vi "Display Images_.vi"(0 "fpga interface in":refnum<k20>, 1 "'stop' notifier":refnum<notifier>, 3 "measure call context in":refnum<class "Measure Call Context.lvclass">, 11 "error in (no error)":errorcluster, 12 "References":T1) -> (4 "fpga interface out":refnum<k20>, 15 "error out":errorcluster)   [LabVIEW 2025, in "GettingStarted_Common_148X_Host.lvlib"]
uses:
  GettingStarted_Common_148X_Host.lvlib
  <vilib>/Plug-In SDKs/Measurements/Measure Call Context/Measure Call Context.lvclass
  Types/148x_Common_FPGA_Reference.ctl
  <instrlib>/FlexRIO/CSI-2/v2/Common/Types/LLP Data Type.ctl
  Measurement Results.ctl
  <vilib>/Utility/error.llb/Error Cluster From Error Code.vi
  <vilib>/rvi/errors/niLvFpgaAdjustHostInterfaceError.vi
  <vilib>/rvi/interface/nirviReadWriteControl/nirviReadWriteControl.xnode
  NiFpgaLv.dll
  <vilib>/rvi/interface/Simulation/niFpgaSimulationCallBeginRW.vi
  Automotive Vision.lvclass
  <instrlib>/FlexRIO/CSI-2/v2/Common/NI CSI-2 API Common v2.lvlib
panel:
  in  "Image decimation":u32=5
  in  "Decimate image":bool
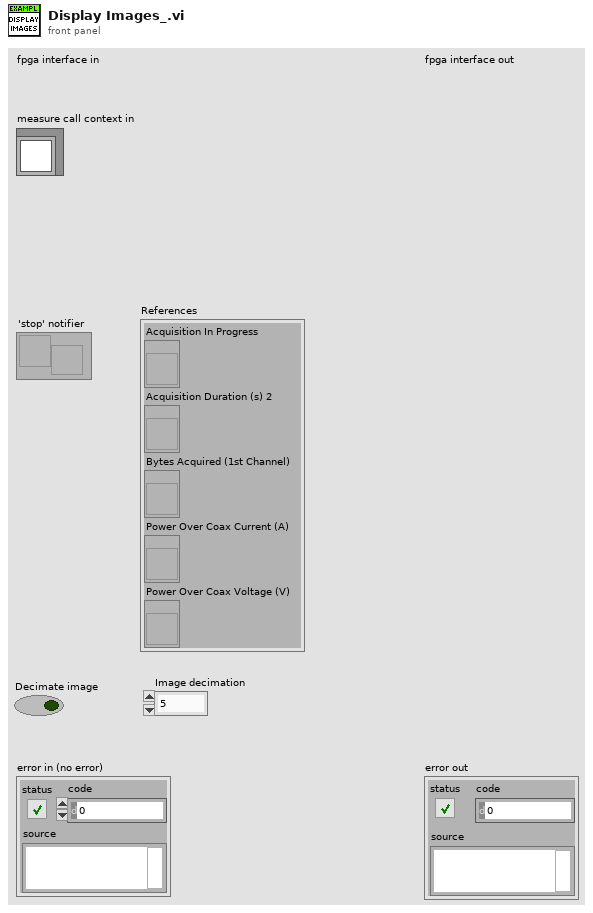
[diagram p1: front panel]
types:
  T1 = cluster{"Acquisition In Progress":refnum<vi>, "Acquisition Duration (s) 2":refnum<vi>, "Bytes Acquired (1st Channel)":refnum<vi>, "Power Over Coax Current (A)":refnum<vi>, "Power Over Coax Voltage (V)":refnum<vi>}
  T2 = typedef "NI CSI-2 API Common v2.lvlib/LLP Data Type.ctl" = enum8{"Frame Start", "Frame End", "Line Start", "Line End", "End of Transmission", "Reserved 0", "Reserved 1", "Reserved 2", "Generic Short Packet 1", "Generic Short Packet 2", "Generic Short Packet 3", "Generic Short Packet 4", "Generic Short Packet 5", "Generic Short Packet 6", "Generic Short Packet 7", "Generic Short Packet 8", "Null", "Blanking Data", "Embedded 8-bit non Image Data", "Generic Long Packet 1", "Generic Long Packet 2", "Generic Long Packet 3", "Generic Long Packet 4", "Reserved 3", "YUV420 8-bit", "YUV420 10-bit", "Legacy YUV420 8-bit", "Reserved 4", "YUV420 8-bit Chroma Shifted", "YUV420 10-bit Chroma Shifted", "YUV422 8-bit", "YUV422 10-bit", "RGB444", "RGB555", "RGB565", "RGB666", "RGB888", "Reserved 5", "Reserved 6", "RAW 24", "RAW 6", "RAW 7", "RAW 8", "RAW 10", "RAW 12", "RAW 14", "RAW 16", "RAW 20", "User Defined 8-bit Data 1", "User Defined 8-bit Data 2", "User Defined 8-bit Data 3", "User Defined 8-bit Data 4", "User Defined 8-bit Data 5", "User Defined 8-bit Data 6", "User Defined 8-bit Data 7", "User Defined 8-bit Data 8", "USL Command", "Reserved 7", "Reserved 8", "Reserved 9", "Reserved 10", "Reserved 11", "Reserved 12", "LRTE EPD Spacer"}
  T3 = cluster{"serial channel":fxp<+,3,3>, "frame number":u16, "data type":T2, "width":u16, "height":u16, "image bytes":u32, "total bytes":u32, "little endian":bool, "Status":string}
  T4 = typedef "GettingStarted_Common_148X_Host.lvlib/148x_Common_FPGA_Reference.ctl" = refnum<k20>
  T5 = typedef "Automotive Vision.lvclass/Measurement Results.ctl" = cluster{"ACQ. IN PROGRESS":bool, "Array":u32[], "ACQ. DURATION (s)":dbl, "SOURCE RATE (fps)":dbl, "BYTES ACQUIRED":u64, "FRAME COUNT":u64, "POC VOLTAGE (V)":dbl, "POC CURRENT (A)":dbl, "ERROR":bool, "STATE MESSAGE":string, "IMAGE DATA":string, "OOB gRPC Port":i32}
  T6 = typedef "GettingStarted_Common_148X_FPGA.lvlib/Image Metadata.ctl" = cluster{"serial channel":fxp<+,3,3>, "frame number":u16, "data type":T2, "width":u16, "height":u16, "image bytes":u32, "total bytes":u32, "little endian":bool}
  T7 = typedef "Automotive-Vision OOB Data Transfer.lvlib/OOB to Logic Data.ctl" = cluster{"PauseResume":bool, "ExportPath":string, "ExportType":u16, "Export":bool}
  T8 = cluster{"image pixel data fifo overflow":bool, "image metadata fifo overflow":bool}[]
  T9 = cluster{"image pixel data fifo overflow":bool, "image metadata fifo overflow":bool}
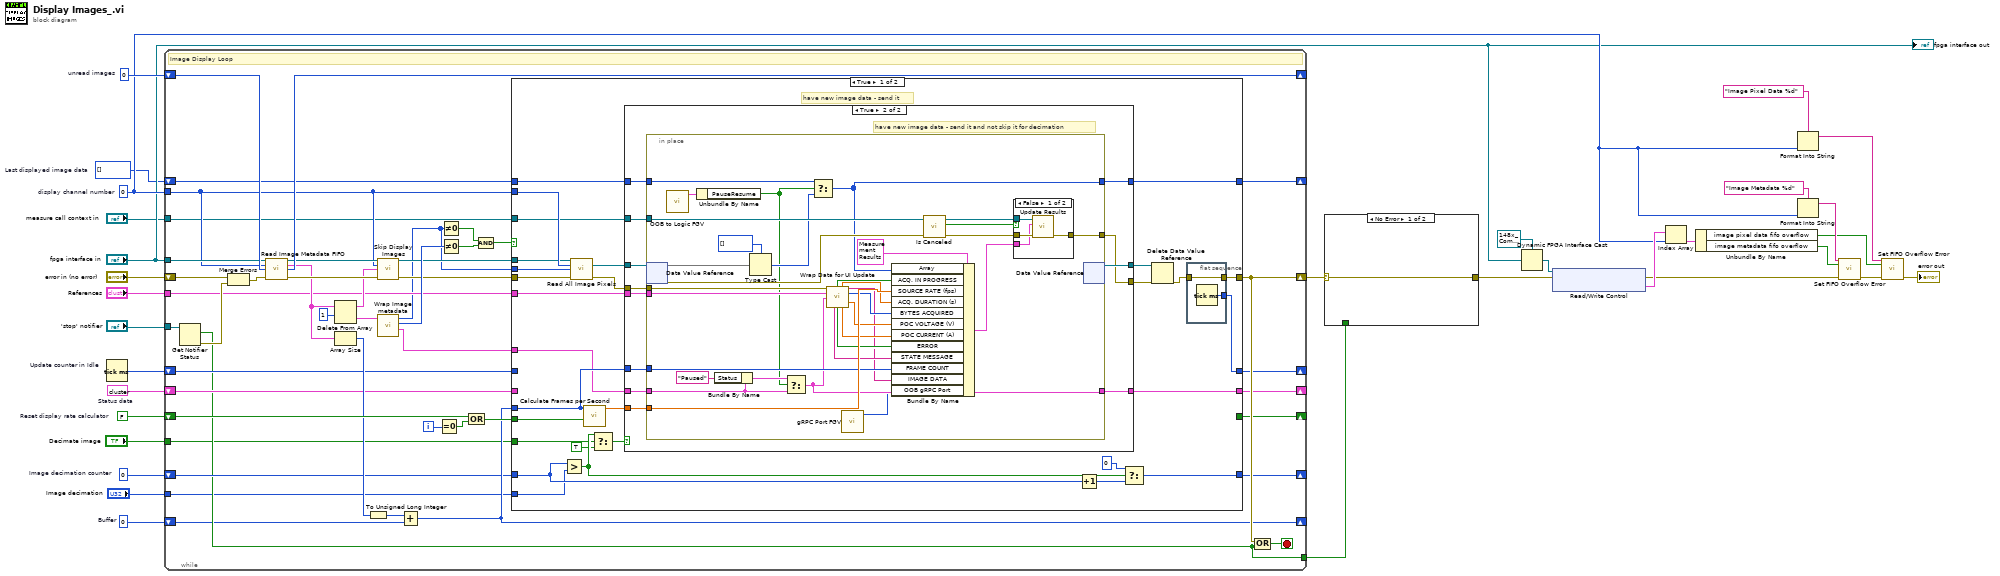
[diagram p0: block diagram]
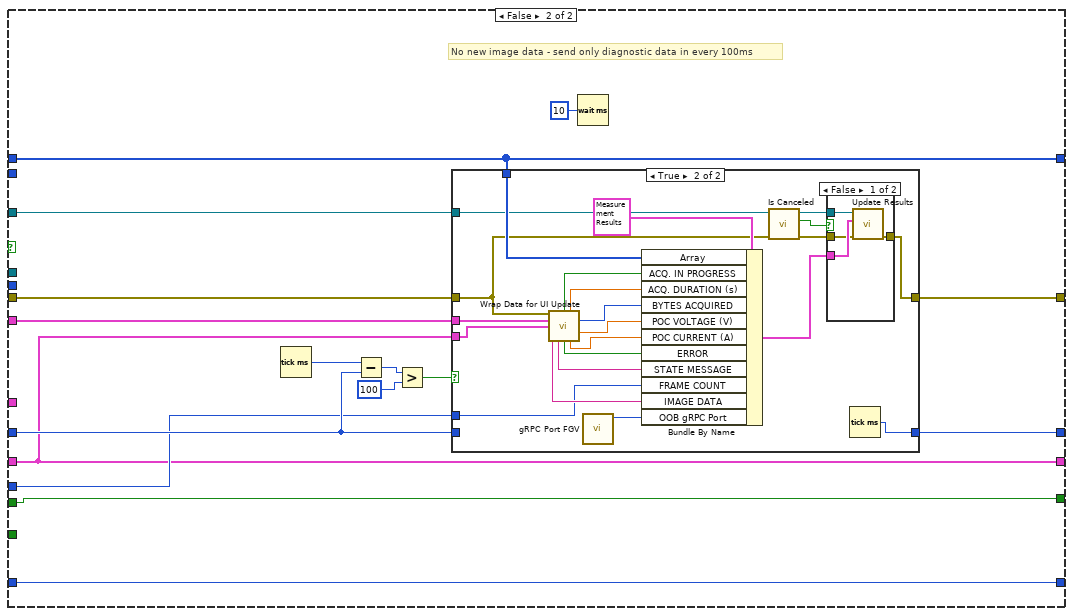
[diagram p4: hidden frame]
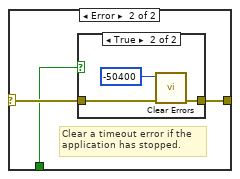
[diagram p7: hidden frame]
diagram:
  w3 = T3 {"serial channel"=0.0, "frame number"=0, "data type"=enum."Frame Start", "width"=0, "height"=0, "image bytes"=0, "total bytes"=0, "little endian"=FALSE, "Status"="Ready for Acquisition"}  # Status data
  w22 = 0  # display channel number
  w7 = u32 0  # Image decimation counter
  w8 = u32[] []  # Last displayed image data
  w14 = u32 0  # Buffer
  w15 = FALSE  # Reset display rate calculator
  w31 = u32 0  # unread images
  n1 = Tick Count (ms) "Update counter in Idle"() -> (millisecond timer value=w9:u32)
  n2 = while {
    shift-right: [w74] -> w13
    shift-left: "error in (no error)" -> [w50]
    tunnel: "fpga interface in" -> [w53]
    shift-right: [w75] -> _
    shift-left: w31 -> [w65]
    tunnel: w22 -> [w49]
    shift-right: [w69] -> _
    shift-left: w15 -> [w66]
    shift-right: [w55] -> _
    shift-left: w14 -> [w32]
    tunnel: [w36] -> w11
    tunnel: "'stop' notifier" -> [w52]
    shift-right: [w47] -> _
    shift-left: w9 -> [w48]
    shift-right: [w45] -> _
    shift-left: w8 -> [w46]
    shift-right: [w43] -> _
    shift-left: w7 -> [w44]
    tunnel: "References" -> [w42]
    tunnel: "measure call context in" -> [w41]
    shift-right: [w39] -> _
    shift-left: w3 -> [w40]
    tunnel: "Image decimation" -> [w35]
    tunnel: "Decimate image" -> [w34]
    i -> [w73]
    stop <- w76 stop-if-true
    # "Image Display Loop"
    n3 = Get Notifier Status(notifier=w52) -> (current notification=w36:bool, error out=w77:errorcluster)  [unwired: 1 in, 3 out]
    n4 = Merge Errors(w50, w77) -> (w51:errorcluster)
    n5 = call "Read Image Metadata FIFO.vi"("fpga inteface in"=w53, "display channel number"=w49, "number of images"=w65, "error in (no error)"=w51) -> ("fpga interface out"=w61:refnum<k20>, "image metadata"=w54:T6[], "images remaining"=w75:u32, "error out"=w58:errorcluster)  [unwired: 8 in]
    n6 = Delete From Array(array=w54, length=1) -> (deleted portion=w62:T6[], array with subset deleted=w57:T6[])  [unwired: 1 in]
    n7 = Array Size(array=w54) -> (size(s)=w56:i32)
    n8 = To Unsigned Long Integer(number=w56) -> (unsigned 32bit integer=w33:u32)
    n9 = call "Skip Display Images.vi"("fpga interface in"=w61, "display channel number"=w49, "image metadata"=w57, "error in (no error)"=w58) -> ("fpga interface out"=w60:refnum<k20>, "error out"=w59:errorcluster)  [unwired: 10 in]
    n10 = call "Wrap Image metadata.vi"("image metadata"=w62) -> ("element"=w38:T3, "Numeric"=w64:i32, "total bytes"=w37:u32)  [unwired: 8 in]
    n11 = Add(x=w33, y=w32) -> (x+y=w55:u32)
    n12 = Equal To 0?(x=w73) -> (x = 0?=w67:bool)
    n13 = Not Equal To 0?(x=w37) -> (x != 0?=w71:bool)
    n14 = Not Equal To 0?(x=w64) -> (x != 0?=w72:bool)
    n15 = Compound Arithmetic op=OR(w66, w67) -> (w68:bool)
    n16 = Compound Arithmetic op=AND(w71, w72) -> (w70:bool)
    n17 = case shown="True" w70 {
      tunnel: w59 -> [w102 w162]
      tunnel: w60 -> [w105 _]
      tunnel: w49 -> [w106 _]
      tunnel: [w96 w169] -> w74
      tunnel: w68 -> [w81 w176]
      tunnel: [_ w176] -> w69
      tunnel: w55 -> [w93 w166]
      tunnel: w37 -> [w100 _]
      tunnel: w38 -> [w84 _]
      tunnel: w41 -> [w98 w163]
      tunnel: w42 -> [w97 w177]
      tunnel: w48 -> [_ w168]
      tunnel: [w95 w170] -> w47
      tunnel: w46 -> [w92 w167]
      tunnel: [w94 w167] -> w45
      tunnel: w44 -> [w90 w165]
      tunnel: [w88 w165] -> w43
      tunnel: w40 -> [_ w164]
      tunnel: [w83 w164] -> w39
      tunnel: w35 -> [w79 _]
      tunnel: w34 -> [w78 _]
      frame True {
        # "have new image data - send it"
        n18 = Greater?(x=w90, y=w79) -> (0:w87:bool)
        n19 = call "Read All Image Pixels.vi"("fpga inteface in"=w105, "display channel number"=w106, "image bytes"=w100, "error in (no error)"=w102) -> ("image pixel data region"=w104:refnum<data-value>, "error out"=w99:errorcluster)  [unwired: 8 in, 2 out]
        n20 = call <vilib>:"Calculate Frames per Second.vi"("Reset"=w81, "Buffer Number"=w93) -> ("Acquired Frames/s"=w80:dbl)  [unwired: 7 in, 2 out]
        n21 = Select(t=w87, s=w78, f=TRUE) -> (s? t:f=w86:bool)
        n22 = case shown="True" w86 {
          tunnel: w104 -> [w110 w122]
          tunnel: [w110 w121] -> w103
          tunnel: [w108 w120] -> w101
          tunnel: w80 -> [_ w119]
          tunnel: w99 -> [w108 w118]
          tunnel: w84 -> [w107 w117]
          tunnel: w98 -> [_ w116]
          tunnel: w97 -> [_ w115]
          tunnel: [w109 w114] -> w94
          tunnel: w93 -> [_ w113]
          tunnel: w92 -> [w109 w112]
          tunnel: [w107 w111] -> w83
          frame False {
            # "have new image data - but skip the sending to not overload UI with data transfer"
          }
          frame True {
            # "have new image data - send it and not skip it for decimation"
            n23 = in-place {
              in-place-border: [w150] -> w120
              in-place-border: w119 -> [w149]
              in-place-border: w118 -> [w148]
              in-place-border: w117 -> [w147]
              in-place-border: w116 -> [w146]
              in-place-border: w115 -> [w145]
              in-place-border: [w144] -> w114
              in-place-border: w113 -> [w143]
              in-place-border: w112 -> [w142]
              in-place-border: [w141] -> w111
              n24 = in-place-dvr #1(w122) -> (w151:u8[], w153:errorcluster)
              n25 = call "OOB to Logic FGV.vi"() -> ("OOB to Logic Data out"=w124:T7)  [unwired: 10 in, 1 out]
              n26 = Unbundle By Name(w124) -> ("PauseResume"=w123:bool)
              n27 = Bundle By Name(cluster=w147, "Status"="Paused") -> (w128:T3)
              n28 = Type Cast(type=u32[] [], x=w151) -> (*(type *) &x=w129:u32[])
              n29 = Select(t=w128, s=w123, f=w147) -> (s? t:f=w141:T3)
              n30 = Select(t=w142, s=w123, f=w129) -> (s? t:f=w144:u32[])
              n31 = call "Wrap Data for UI Update.vi"("error in (no error)"=w148, "References"=w145, "image metadata"=w141) -> ("Acqusition In Progress"=w137:bool, "Acquisition Duration"=w136:dbl, "Image Data"=w130:string, "Bytes Acquired"=w135:i64, "PowerOverCoaxCurrent"=w134:dbl, "State message"=w131:string, "status"=w132:bool, "PowerOverCoaxVoltage"=w133:dbl)  [unwired: 4 in, 1 out]
              n32 = call "gRPC Port FGV.vi"() -> ("Listening Port out"=w125:i32)  [unwired: 11 in]
              n33 = Bundle By Name(cluster=T5 {"ACQ. IN PROGRESS"=FALSE, "Array"=[], "ACQ. DURATION (s)"=0.0, "SOURCE RATE (fps)"=0.0, "BYTES ACQUIRED"=0, "FRAME COUNT"=0, "POC VOLTAGE (V)"=0.0, "POC CURRENT (A)"=0.0, "ERROR"=FALSE, "STATE MESSAGE"="", "IMAGE DATA"="", "OOB gRPC Port"=0} ("Measurement Results"), "Array"=w144, "ACQ. IN PROGRESS"=w137, "SOURCE RATE (fps)"=w149, "ACQ. DURATION (s)"=w136, "BYTES ACQUIRED"=w135, "POC VOLTAGE (V)"=w134, "POC CURRENT (A)"=w133, "ERROR"=w132, "STATE MESSAGE"=w131, "FRAME COUNT"=w143, "IMAGE DATA"=w130, "OOB gRPC Port"=w125) -> (w139:T5)
              n34 = call <vilib>:"Is Canceled.vi"("error in"=w153, "measure call context in"=w146) -> ("error out"=w152:errorcluster, "is canceled?"=w126:bool, "measure call context out"=w154:refnum<class "Measure Call Context.lvclass">)  [unwired: 7 in]
              n35 = case shown="False" w126 {
                tunnel: w154 -> [w158 _]
                tunnel: w152 -> [w157 w159]
                tunnel: [w156 w159] -> w150
                tunnel: w139 -> [w155 _]
                frame False {
                  n36 = call <vilib>:"Update Results.vi"("error in"=w157, "measurement results"=w155, "measure call context in"=w158) -> ("error out"=w156:errorcluster)  [unwired: 7 in, 1 out]
                }
                frame True {
                }
              }
              n37 = in-place-dvr #1() -> (w121:refnum<data-value>)  [unwired: 1 in, 1 out]
            }
          }
        }
        n38 = Increment(x=w90) -> (x+1=w89:u32)
        n39 = Select(t=u32 0 ("y"), s=w87, f=w89) -> (s? t:f=w88:u32)
        n40 = Delete Data Value Reference(data value reference=w103, error in=w101) -> (error out=w82:errorcluster)  [unwired: 1 out]
        n41 = flat-sequence {
          tunnel: [w161] -> w96
          tunnel: w82 -> [w161]
          tunnel: [w160] -> w95
          frame #0 {
            n42 = Tick Count (ms)() -> (millisecond timer value=w160:u32)
          }
        }
      }
      frame False {
        # "No new image data - send only diagnostic data in every 100ms"
        n43 = Tick Count (ms)() -> (millisecond timer value=w174:u32)
        n44 = Subtract(x=w174, y=w168) -> (x-y=w173:u32)
        n45 = Greater?(x=w173, y=u32 100) -> (0:w171:bool)
        n46 = case shown="True" w171 {
          tunnel: w162 -> [w179 w181]
          tunnel: [w179 w199] -> w169
          tunnel: w164 -> [_ w186]
          tunnel: w177 -> [_ w187]
          tunnel: [w178 w190] -> w170
          tunnel: w168 -> [w178 _]
          tunnel: w167 -> [_ w189]
          tunnel: w166 -> [_ w188]
          tunnel: w163 -> [_ w185]
          frame False {
          }
          frame True {
            n47 = call "Wrap Data for UI Update.vi"("error in (no error)"=w181, "References"=w187, "image metadata"=w186) -> ("Acqusition In Progress"=w198:bool, "Acquisition Duration"=w197:dbl, "Image Data"=w191:string, "Bytes Acquired"=w196:i64, "PowerOverCoaxCurrent"=w195:dbl, "State message"=w192:string, "status"=w193:bool, "PowerOverCoaxVoltage"=w194:dbl)  [unwired: 4 in, 1 out]
            n48 = call "gRPC Port FGV.vi"() -> ("Listening Port out"=w180:i32)  [unwired: 11 in]
            n49 = Bundle By Name(cluster=T5 {"ACQ. IN PROGRESS"=FALSE, "Array"=[], "ACQ. DURATION (s)"=0.0, "SOURCE RATE (fps)"=0.0, "BYTES ACQUIRED"=0, "FRAME COUNT"=0, "POC VOLTAGE (V)"=0.0, "POC CURRENT (A)"=0.0, "ERROR"=FALSE, "STATE MESSAGE"="", "IMAGE DATA"="", "OOB gRPC Port"=0} ("Measurement Results"), "Array"=w189, "ACQ. IN PROGRESS"=w198, "ACQ. DURATION (s)"=w197, "BYTES ACQUIRED"=w196, "POC VOLTAGE (V)"=w195, "POC CURRENT (A)"=w194, "ERROR"=w193, "STATE MESSAGE"=w192, "FRAME COUNT"=w188, "IMAGE DATA"=w191, "OOB gRPC Port"=w180) -> (w200:T5)
            n50 = call <vilib>:"Is Canceled.vi"("error in"=w181, "measure call context in"=w185) -> ("error out"=w182:errorcluster, "is canceled?"=w183:bool, "measure call context out"=w184:refnum<class "Measure Call Context.lvclass">)  [unwired: 7 in]
            n51 = case shown="False" w183 {
              tunnel: w200 -> [w205 _]
              tunnel: [w204 w206] -> w199
              tunnel: w184 -> [w203 _]
              tunnel: w182 -> [w202 w206]
              frame False {
                n52 = call <vilib>:"Update Results.vi"("error in"=w202, "measurement results"=w205, "measure call context in"=w203) -> ("error out"=w204:errorcluster)  [unwired: 7 in, 1 out]
              }
              frame True {
              }
            }
            n53 = Tick Count (ms)() -> (millisecond timer value=w190:u32)
          }
        }
        n54 = Wait (ms)(milliseconds to wait=u32 10) -> ()  [unwired: 1 out]
      }
    }
    n55 = Compound Arithmetic op=OR(w74, w36) -> (w76:bool)
  }
  n56 = case shown="No Error" w13 {
    selector: w13 -> [w207 w210]
    tunnel: [w207 w209] -> w26
    tunnel: w11 -> [_ w208]
    frame No Error {
    }
    frame Error {
      # "Clear a timeout error if the application has stopped."
      n57 = case shown="True" w208 {
        tunnel: w210 -> [w211 w214]
        tunnel: [w211 w212] -> w209
        frame False {
        }
        frame True {
          n58 = call <vilib>:"Clear Errors.vi"("error in (no error)"=w214, "specific error code to clear (0: all)"=-50400 ("y")) -> ("error out"=w212:errorcluster)  [unwired: 4 in, 1 out]
        }
      }
    }
  }
  n59 = Dynamic FPGA Interface Cast(Session In=T4 refnum ("FPGA VI Reference Out"), Type="fpga interface in") -> (Session Out=w27:T4)
  n60 = xnode "Read/Write Control"("FPGA VI Reference In"=w27, "error in"=w26) -> ("error out"=w25:errorcluster, "display channel status"=w29:T8)  [unwired: 1 out]
  n61 = Index Array(array=w29, index=w22) -> (element=w30:T9)
  n62 = Unbundle By Name(w30) -> ("image pixel data fifo overflow"=w17:bool, "image metadata fifo overflow"=w16:bool)
  n63 = Format Into String(format string="Image Pixel Data %d", w22) -> (resulting string=w19:string)  [unwired: 2 in, 1 out]
  n64 = Format Into String(format string="Image Metadata %d", w22) -> (resulting string=w18:string)  [unwired: 2 in, 1 out]
  n65 = call "Set FIFO Overflow Error.vi"("fifo name"=w18, "overflow"=w16, "error in (no error)"=w25) -> ("error out"=w21:errorcluster)  [unwired: 12 in]
  n66 = call "Set FIFO Overflow Error.vi"("fifo name"=w19, "overflow"=w17, "error in (no error)"=w21) -> ("error out"=→"error out":errorcluster)  [unwired: 12 in]
  "fpga interface out" <- "fpga interface in"
